vi "Get TS Variables.vi"(8 "error in (no error)":errorcluster, 11 "Sequence Context In":refnum<k7>) -> (0 "error out":errorcluster, 2 "Variables":T1 {"Tx Values In" format="%.2f"}, 3 "Sequence Context Out":refnum<k7>)   [LabVIEW 2019, in "Wrappers.lvlib"]
uses:
  Wrappers.lvlib
  <vilib>/addons/TestStand/_TSUtility.llb/TestStand - Get Property Value (Boolean).vi
  <vilib>/addons/TestStand/_TSUtility.llb/TestStand - Get Property Value (String Array).vi
  <vilib>/addons/TestStand/_TSUtility.llb/TestStand - Get Property Value (Numeric Array).vi
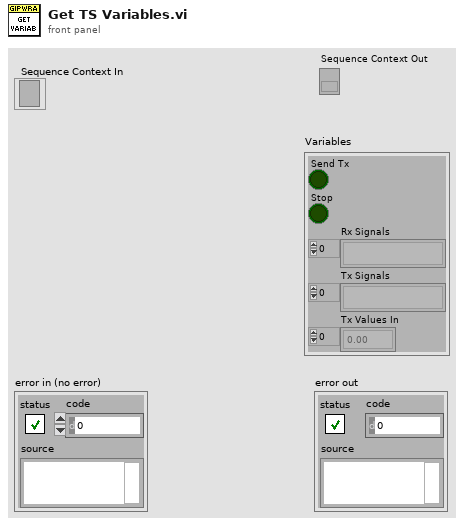
[diagram p1: front panel]
types:
  T1 = cluster{"Send Tx":bool, "Stop":bool, "Rx Signals":string[], "Tx Signals":string[], "Tx Values In":dbl[]}
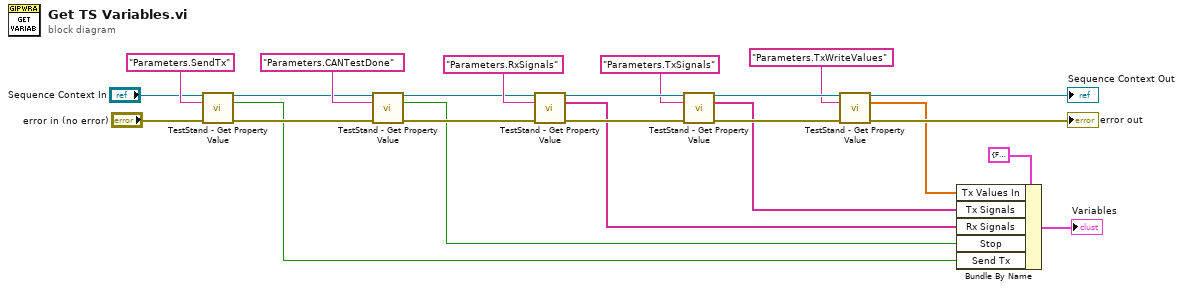
[diagram p0: block diagram]
diagram:
  n1 = call-poly <vilib>:"TestStand - Get Property Value.vi"("Sequence Context In"="Sequence Context In", "Lookup String"="Parameters.SendTx", "error in (no error)"="error in (no error)") -> ("Sequence Context Out"=w11:refnum<k7>, "Value"=w6:bool, "error out"=w9:errorcluster)  [unwired: 10 in]
  n2 = call-poly <vilib>:"TestStand - Get Property Value.vi"("Sequence Context In"=w11, "Lookup String"="Parameters.CANTestDone", "error in (no error)"=w9) -> ("Sequence Context Out"=w10:refnum<k7>, "Value"=w5:bool, "error out"=w8:errorcluster)  [unwired: 10 in]
  n3 = call-poly <vilib>:"TestStand - Get Property Value.vi"("Sequence Context In"=w10, "Lookup String"="Parameters.RxSignals", "error in (no error)"=w8) -> ("Sequence Context Out"=w20:refnum<k7>, "Value"=w4:string[], "error out"=w21:errorcluster)  [unwired: 10 in]
  n4 = call-poly <vilib>:"TestStand - Get Property Value.vi"("Sequence Context In"=w20, "Lookup String"="Parameters.TxSignals", "error in (no error)"=w21) -> ("Sequence Context Out"=w16:refnum<k7>, "Value"=w3:string[], "error out"=w17:errorcluster)  [unwired: 10 in]
  n5 = call-poly <vilib>:"TestStand - Get Property Value.vi"("Sequence Context In"=w16, "Lookup String"="Parameters.TxWriteValues", "error in (no error)"=w17) -> ("Sequence Context Out"=→"Sequence Context Out":refnum<k7>, "Value"=w2:dbl[], "error out"=→"error out":errorcluster)  [unwired: 10 in]
  n6 = Bundle By Name(cluster=T1 {"Send Tx"=FALSE, "Stop"=FALSE, "Rx Signals"=[], "Tx Signals"=[], "Tx Values In"=[]} ("Variables"), "Tx Values In"=w2, "Tx Signals"=w3, "Rx Signals"=w4, "Stop"=w5, "Send Tx"=w6) -> (→"Variables":T1)
